vi "Response Class Type.vi"(11 "Type":string) -> (3 "Class":refnum<class "Response.lvclass">)   [LabVIEW 2020, in "obs-websocket.lvlib"]
uses:
  obs-websocket.lvlib
  RGetSourceScreenshot/RGetSourceScreenshot.lvclass
  C:/dev/lv20CE/relink/lv-obs-websocket/obs-websocket/Response/Response.lvclass
  RGetSceneList/RGetSceneList.lvclass
  RGetCurrentProgramScene/RGetCurrentProgramScene.lvclass
  RGetStreamStatus/RGetStreamStatus.lvclass
  RGetInputKindList/RGetInputKindList.lvclass
  RGetInputList/RGetInputList.lvclass
  RJSONDebug/RJSONDebug.lvclass
  RGetInputVolume/RGetInputVolume.lvclass
  REmptyResponse/REmptyResponse.lvclass
  RGetSceneItemID/RGetSceneItemID.lvclass
  RGetSceneItemEnabled/RGetSceneItemEnabled.lvclass
  RGetInputMute/RGetInputMute.lvclass
  C:/dev/lv20CE/relink/lv-obs-websocket/obs-websocket/Server Message/Server Message.lvclass
  C:/dev/lv20CE/relink/lv-obs-websocket/obs-websocket/Message/Message.lvclass
  C:/dev/lv20CE/relink/lv-promises/Promises/Value/Value.lvclass
  C:/dev/lv20CE/relink/lv-obs-websocket/obs-websocket/RJSONDebug/RJSONDebug.lvclass
  C:/dev/lv20CE/relink/lv-obs-websocket/obs-websocket/RGetSourceScreenshot/RGetSourceScreenshot.lvclass
  C:/dev/lv20CE/relink/lv-obs-websocket/obs-websocket/RGetSceneList/RGetSceneList.lvclass
  C:/dev/lv20CE/relink/lv-obs-websocket/obs-websocket/RGetCurrentProgramScene/RGetCurrentProgramScene.lvclass
  C:/dev/lv20CE/relink/lv-obs-websocket/obs-websocket/RGetStreamStatus/RGetStreamStatus.lvclass
  C:/dev/lv20CE/relink/lv-obs-websocket/obs-websocket/RGetInputKindList/RGetInputKindList.lvclass
  C:/dev/lv20CE/relink/lv-obs-websocket/obs-websocket/RGetInputList/RGetInputList.lvclass
  C:/dev/lv20CE/relink/lv-obs-websocket/obs-websocket/RGetInputVolume/RGetInputVolume.lvclass
  C:/dev/lv20CE/relink/lv-obs-websocket/obs-websocket/REmptyResponse/REmptyResponse.lvclass
  C:/dev/lv20CE/relink/lv-obs-websocket/obs-websocket/RGetSceneItemID/RGetSceneItemID.lvclass
  C:/dev/lv20CE/relink/lv-obs-websocket/obs-websocket/RGetSceneItemEnabled/RGetSceneItemEnabled.lvclass
  C:/dev/lv20CE/relink/lv-obs-websocket/obs-websocket/RGetInputMute/RGetInputMute.lvclass
  Response/Response.lvclass
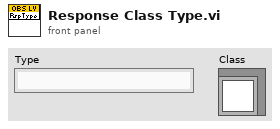
[diagram p1: front panel]
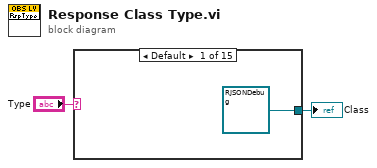
[diagram p0: block diagram]
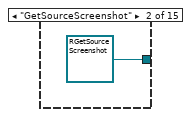
[diagram p2: hidden frame]
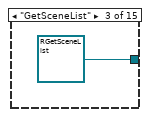
[diagram p3: hidden frame]
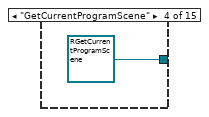
[diagram p4: hidden frame]
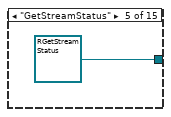
[diagram p5: hidden frame]
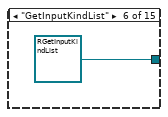
[diagram p6: hidden frame]
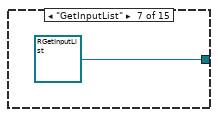
[diagram p7: hidden frame]
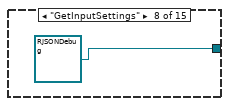
[diagram p8: hidden frame]
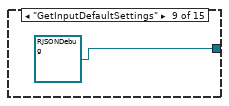
[diagram p9: hidden frame]
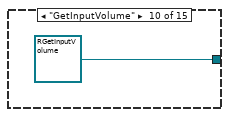
[diagram p10: hidden frame]
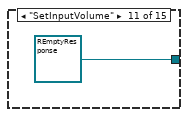
[diagram p11: hidden frame]
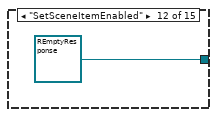
[diagram p12: hidden frame]
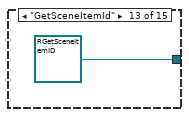
[diagram p13: hidden frame]
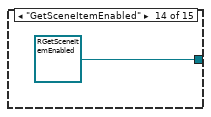
[diagram p14: hidden frame]
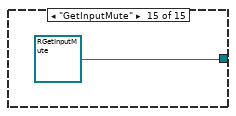
[diagram p15: hidden frame]
diagram:
  n1 = case shown="Default" "Type" {
    tunnel: [refnum<class "RJSONDebug.lvclass"> refnum ("obs-websocket-lv.lvlib:Response.lvclass") refnum<class "RGetSourceScreenshot.lvclass"> refnum ("obs-websocket-lv.lvlib:RGetSourceScreenshot.lvclass") refnum<class "RGetSceneList.lvclass"> refnum ("obs-websocket-lv.lvlib:RGetSceneList.lvclass") refnum<class "RGetCurrentProgramScene.lvclass"> refnum ("obs-websocket-lv.lvlib:RGetCurrentProgramScene.lvclass") refnum<class "RGetStreamStatus.lvclass"> refnum ("obs-websocket-lv.lvlib:RGetStreamStatus.lvclass") refnum<class "RGetInputKindList.lvclass"> refnum ("obs-websocket-lv.lvlib:RJSONDebug.lvclass") refnum<class "RGetInputList.lvclass"> refnum ("obs-websocket-lv.lvlib:RGetInputList.lvclass") refnum<class "RJSONDebug.lvclass"> refnum ("obs-websocket-lv.lvlib:RJSONDebug.lvclass") refnum<class "RJSONDebug.lvclass"> refnum ("obs-websocket-lv.lvlib:RJSONDebug.lvclass") refnum<class "RGetInputVolume.lvclass"> refnum ("obs-websocket-lv.lvlib:RGetInputVolume.lvclass") refnum<class "REmptyResponse.lvclass"> refnum ("obs-websocket-lv.lvlib:REmptyResponse.lvclass") refnum<class "REmptyResponse.lvclass"> refnum ("obs-websocket-lv.lvlib:REmptyResponse.lvclass") refnum<class "RGetSceneItemID.lvclass"> refnum ("obs-websocket-lv.lvlib:RGetSceneItemID.lvclass") refnum<class "RGetSceneItemEnabled.lvclass"> refnum ("obs-websocket-lv.lvlib:RGetSceneItemEnabled.lvclass") refnum<class "RGetInputMute.lvclass"> refnum ("obs-websocket-lv.lvlib:RGetInputMute.lvclass")] -> w1
    frame Default {
    }
    frame "GetSourceScreenshot" {
    }
    frame "GetSceneList" {
    }
    frame "GetCurrentProgramScene" {
    }
    frame "GetStreamStatus" {
    }
    frame "GetInputKindList" {
    }
    frame "GetInputList" {
    }
    frame "GetInputSettings" {
    }
    frame "GetInputDefaultSettings" {
    }
    frame "GetInputVolume" {
    }
    frame "SetInputVolume" {
    }
    frame "SetSceneItemEnabled" {
    }
    frame "GetSceneItemId" {
    }
    frame "GetSceneItemEnabled" {
    }
    frame "GetInputMute" {
    }
  }
  "Class" <- w1
